vi "calculate offset.vi"(1 "outpin in":sgl, 2 "Calculate offset":bool, 3 "avg of":i32, 4 "numeric array":sgl[](array[numeric])) -> (0 "Offset":sgl)   [LabVIEW 2019]
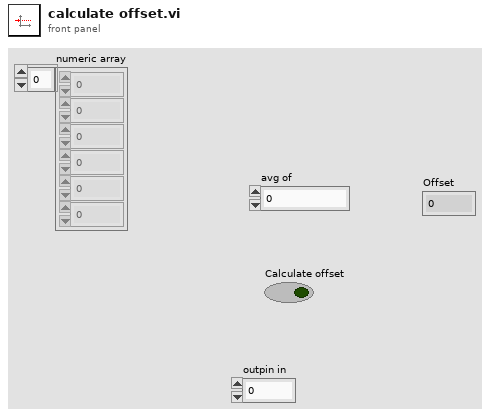
[diagram p1: front panel]
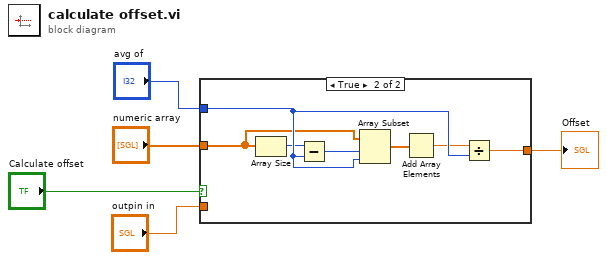
[diagram p0: block diagram]
diagram:
  n1 = case shown="True" "Calculate offset" {
    tunnel: "avg of" -> [_ w13]
    tunnel: [w6 w12] -> w4
    tunnel: "numeric array" -> [_ w11]
    tunnel: "outpin in" -> [w6 _]
    frame False {
    }
    frame True {
      n2 = Array Size(array=w11) -> (size(s)=w9:i32)
      n3 = Subtract(x=w9, y=w13) -> (x-y=w8:i32)
      n4 = Array Subset(array=w11, index=w8, length=w13) -> (w7:sgl[])
      n5 = Add Array Elements(numeric array=w7) -> (sum=w10:sgl)
      n6 = Divide(x=w10, y=w13) -> (x/y=w12:sgl)
    }
  }
  "Offset" <- w4
